vi "Initialize Channel Editor State.vi"(8 "error in (no error)":errorcluster, 11 "Routing Channel Ref in":T5 format="%.0x") -> (0 "error out":errorcluster, 2 "Channel Editor State":T1, 3 "Routing Channel Ref out":T5 format="%.0x")   [LabVIEW 2017, in "Routing and Faulting System Explorer.lvlib"]
uses:
  Routing and Faulting System Explorer.lvlib
  <vilib>/NI Veristand/Custom Device API/Custom Device Item Ref.ctl
  Channel Editor State.ctl
  Shared/Routing and Faulting Hardware API/Types/Possible Connections for Endpoint.ctl
  Shared/Alias Mapping.ctl
  Alias Map by Module.ctl
  <vilib>/NI VeriStand/Custom Device API/Custom Device API.lvlib
  Shared/Routing and Faulting Shared.lvlib
  Shared/Routing and Faulting Hardware API/Routing and Faulting Hardware API.lvlib
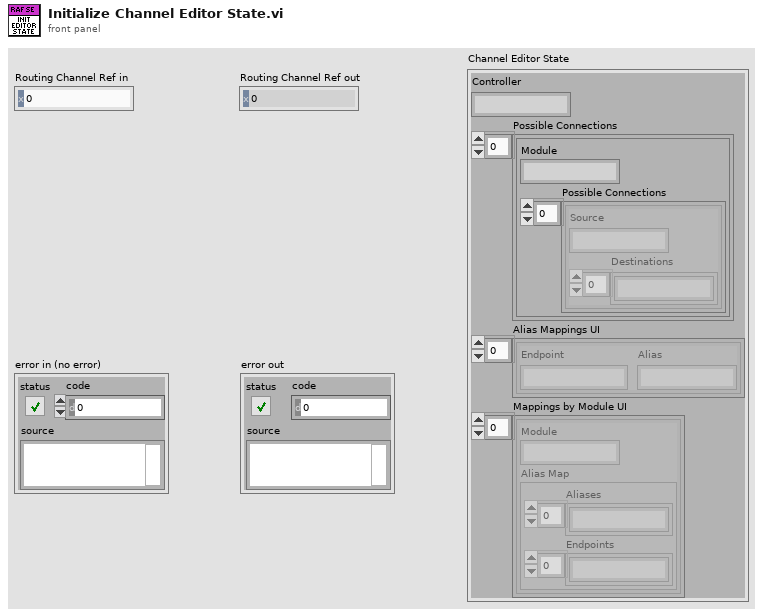
[diagram p1: front panel]
types:
  T1 = typedef "Routing and Faulting System Explorer.lvlib/Channel Editor State.ctl" = cluster{"Controller":string, "Possible Connections":cluster{"Module":string, "Possible Connections":T2[]}[], "Alias Mappings UI":T3[], "Mappings by Module UI":T4[]}
  T2 = typedef "Routing and Faulting Hardware API.lvlib/Possible Connections for Endpoint.ctl" = cluster{"Source":string, "Destinations":string[]}
  T3 = typedef "Routing and Faulting Shared.lvlib/Alias Mapping.ctl" = cluster{"Endpoint":string, "Alias":string}
  T4 = typedef "Routing and Faulting System Explorer.lvlib/Alias Map by Module.ctl" = cluster{"Module":string, "Alias Map":cluster{"Aliases":string[], "Endpoints":string[]}}
  T5 = typedef "Custom Device API.lvlib/Custom Device Item Ref.ctl" = u64
  T6 = cluster{"Controller":string, "Possible Connections":cluster{"Module":string, "Possible Connections":T2[]}[], "Alias Mappings UI":T3[], "Mappings by Module UI":T4[]}
  T7 = typedef "Custom Device API.lvlib/Custom Device Item Info.ctl" = cluster{"Name":string, "Is Channel":bool, "GUID":string, "Is Waveform":bool}
  T8 = cluster{"Module":string, "Possible Connections":T2[]}[]
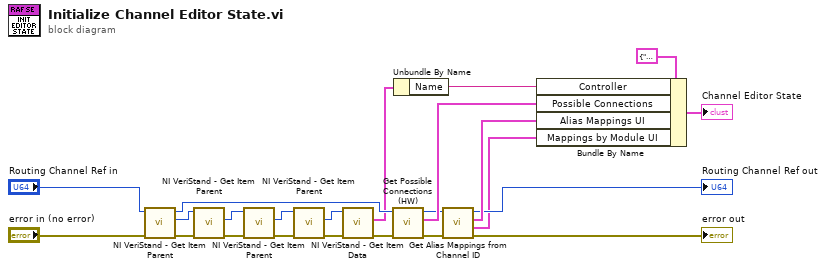
[diagram p0: block diagram]
diagram:
  n1 = call <vilib>:"NI VeriStand - Get Item Parent.vi"("error in (no error)"="error in (no error)", "Item Ref in"="Routing Channel Ref in") -> ("error out"=w22:errorcluster, "Parent Ref"=w23:T5, "Item Ref out"=w12:T5)  [unwired: 6 in, 1 out]
  n2 = call <vilib>:"NI VeriStand - Get Item Parent.vi"("error in (no error)"=w22, "Item Ref in"=w23) -> ("error out"=w20:errorcluster, "Parent Ref"=w7:T5)  [unwired: 6 in, 2 out]
  n3 = call <vilib>:"NI VeriStand - Get Item Parent.vi"("error in (no error)"=w20, "Item Ref in"=w7) -> ("error out"=w21:errorcluster, "Parent Ref"=w8:T5)  [unwired: 6 in, 2 out]
  n4 = call <vilib>:"NI VeriStand - Get Item Parent.vi"("error in (no error)"=w21, "Item Ref in"=w8) -> ("error out"=w4:errorcluster, "Parent Ref"=w5:T5)  [unwired: 6 in, 2 out]
  n5 = call <vilib>:"NI VeriStand - Get Item Data.vi"("error in (no error)"=w4, "Item Ref in"=w5) -> ("error out"=w3:errorcluster, "Item Info"=w6:T7)  [unwired: 6 in, 2 out]
  n6 = call "Get Possible Connections (HW).vi"("error in (no error)"=w3, "Routing Channel Ref in"=w12) -> ("error out"=w18:errorcluster, "Possible Connections"=w16:T8, "Routing Channel Ref out"=w11:T5)  [unwired: 7 in]
  n7 = Unbundle By Name(w6) -> ("Name"=w2:string)
  n8 = call "Get Alias Mappings from Channel ID.vi"("error in (no error)"=w18, "Routing Channel Ref in"=w11) -> ("error out"=→"error out":errorcluster, "Mappings by Module UI"=w9:T4[], "Alias Mappings UI"=w15:T3[], "Routing Channel Ref out"=→"Routing Channel Ref out":T5)  [unwired: 6 in]
  n9 = Bundle By Name(cluster=T6 {"Controller"="", "Possible Connections"=[], "Alias Mappings UI"=[], "Mappings by Module UI"=[]} ("Channel Editor State"), "Controller"=w2, "Possible Connections"=w16, "Alias Mappings UI"=w15, "Mappings by Module UI"=w9) -> (→"Channel Editor State":T6)
